vi "Old CAM Run Test.vi"() -> ()   [LabVIEW 2015]
uses:
  <vilib>/rvi/interface/nirviOpenFPGA/nirviOpenFPGA.xnode
  <vilib>/rvi/interface/nirviReadWriteControl/nirviReadWriteControl.xnode
  <vilib>/rvi/interface/Simulation/niFpgaSimulationCallBeginRW.vi
  <vilib>/rvi/errors/niLvFpgaAdjustHostInterfaceError.vi
  <vilib>/rvi/interface/nirviMethod/nirviMethod.xnode
  <vilib>/rvi/interface/nirviCloseFPGA/nirviCloseFPGA.xnode
  NiFpgaLv.dll
  <vilib>/Utility/error.llb/Error Cluster From Error Code.vi
  Compile Tests/old APU + 4 CAMs.vi
  <vilib>/rvi/interface/RandomDataEmulation/nirviRandomDataOpen.vi
  <vilib>/rvi/interface/common/niFpgaCacheSessionInfoDynamic.vi
  <vilib>/FPGAPlugInAG/Dynamic/niLvFpga_Run_Dynamic.vi
  <vilib>/FPGAPlugInAG/Dynamic/niLvFpga_Close_Dynamic.vi
  Data File Loader/AngleReference.ctl
panel:
  in  "Tooth Angles":cluster{"Falling Edge":dbl, "Rising Edge":dbl}[](array[cluster])=[{"Falling Edge"=0.0, "Rising Edge"=360.0}]
  out "Load done":bool
  out "Load time (s)":dbl=1.2129865353927016e-05
  in  "RPM":dbl=500.0 format="%#_15g"
  in  "stop":bool
  in  "acceleration (RPM/sec)":dbl=inf
  in  "CycleAngle?":T1=TRUE
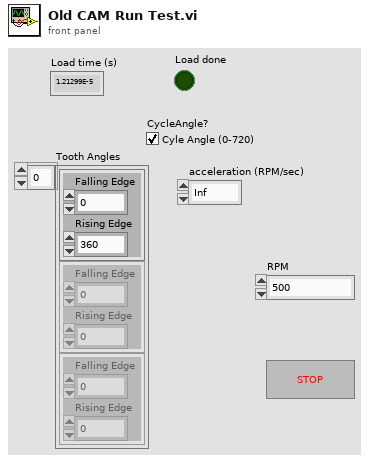
[diagram p1: front panel]
types:
  T1 = typedef "AngleReference.ctl" = bool
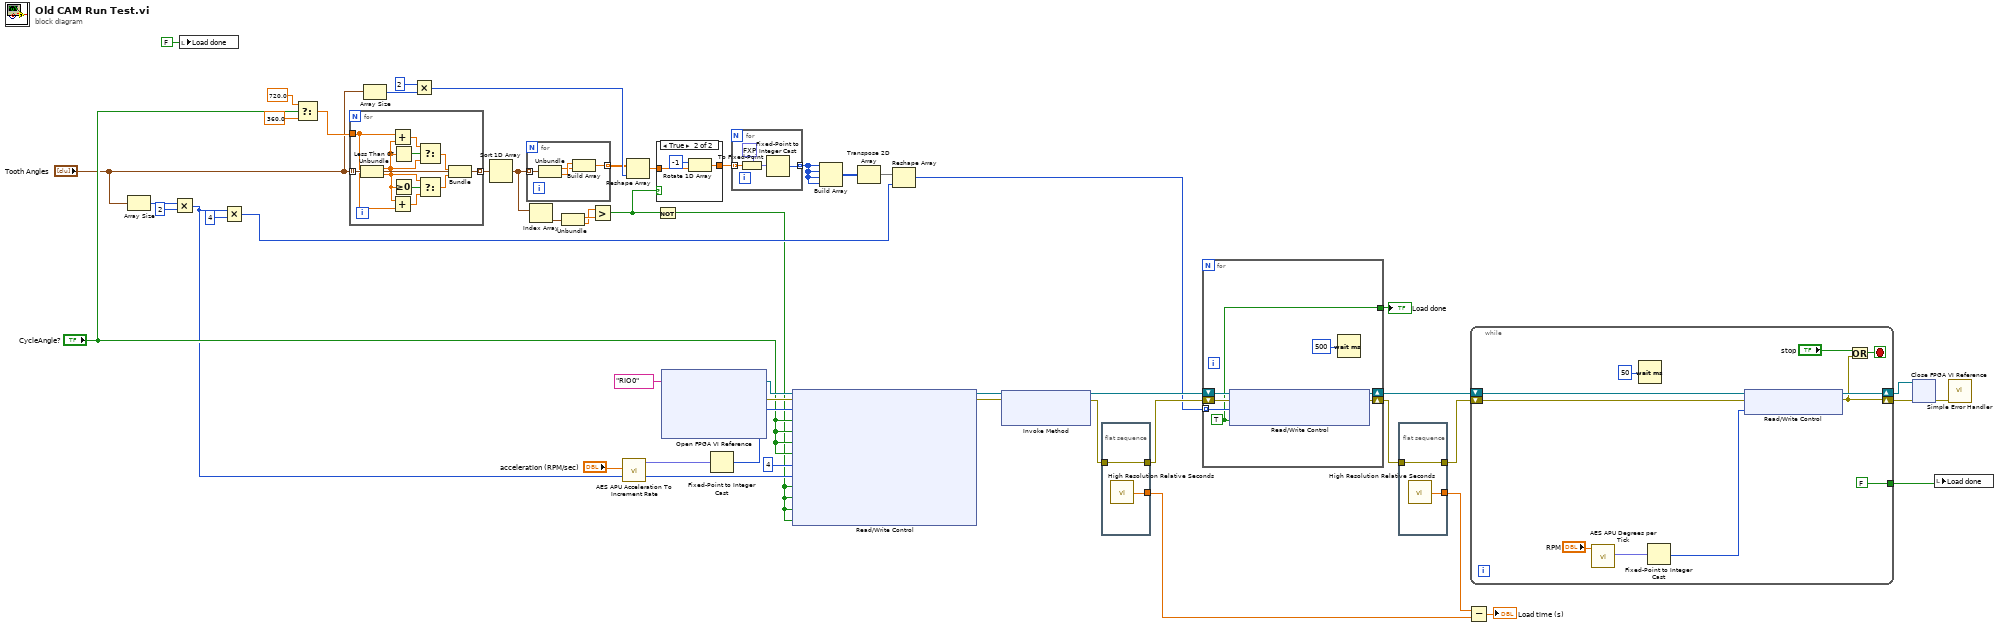
[diagram p0: block diagram]
diagram:
  n1 = Array Size(array="Tooth Angles") -> (size(s)=w11:i32)
  n2 = Multiply(x=w11, y=2) -> (x*y=w6:i32)
  n3 = local write "Load done"(FALSE ("Load done")) -> ()
  n4 = Multiply(x=w6, y=4) -> (x*y=w4:i32)
  n5 = Select(t=720.0 ("y"), s="CycleAngle?", f=360.0) -> (s? t:f=w16:dbl)
  n6 = for {
    tunnel: "Tooth Angles" -> [w56] mode=indexing
    tunnel: [w53] -> w19 mode=indexing
    tunnel: w16 -> [w52]
    n7 = Unbundle(w56) -> ("Falling Edge"=w59:dbl, "Rising Edge"=w57:dbl)
    n8 = Add(x=w52, y=w59) -> (x+y=w60:dbl)
    n9 = Add(x=w57, y=w52) -> (x+y=w58:dbl)
    n10 = Less Than 0?(x=w59) -> (x < 0?=w62:bool)
    n11 = Greater Or Equal To 0?(x=w57) -> (x >= 0?=w61:bool)
    n12 = Select(t=w60, s=w62, f=w59) -> (s? t:f=w55:dbl)
    n13 = Select(t=w57, s=w61, f=w58) -> (s? t:f=w54:dbl)
    n14 = Bundle(cluster=w56, "Falling Edge"=w55, "Rising Edge"=w54) -> (w53:cluster{"Falling Edge":dbl, "Rising Edge":dbl})
  }
  n15 = Array Size(array="Tooth Angles") -> (size(s)=w28:i32)
  n16 = Multiply(x=u16 2, y=w28) -> (x*y=w29:i32)
  n17 = Sort 1D Array(array=w19) -> (sorted array=w21:cluster{"Falling Edge":dbl, "Rising Edge":dbl}[])
  n18 = for {
    tunnel: w21 -> [w66] mode=indexing
    tunnel: [w63] -> w20 mode=indexing
    n19 = Unbundle(w66) -> ("Falling Edge"=w64:dbl, "Rising Edge"=w65:dbl)
    n20 = Build Array(w65, w64) -> (w63:dbl[])
  }
  n21 = Index Array(array=w21) -> (element=w22:cluster{"Falling Edge":dbl, "Rising Edge":dbl})  [unwired: 1 in]
  n22 = Unbundle(w22) -> ("Falling Edge"=w24:dbl, "Rising Edge"=w23:dbl)
  n23 = Greater?(x=w23, y=w24) -> (0:w26:bool)
  n24 = call <userlib>:"AES APU Acceleration To Increment Rate.vi"("acceleration (RPM/sec)"="acceleration (RPM/sec)") -> ("increment rate"=w31:fxp<+/-,47,-4>)  [unwired: 10 in]
  n25 = Reshape Array(w20, w29) -> (w25:dbl[])
  n26 = case shown="True" w26 {
    tunnel: w25 -> [w67 w70]
    tunnel: [w67 w68] -> w18
    frame False {
    }
    frame True {
      n27 = Rotate 1D Array(1:w70, 2:-1 ("n")) -> (0:w68:dbl[])
    }
  }
  n28 = Not(x=w26) -> (.not. x?=w3:bool)
  n29 = xnode "Open FPGA VI Reference"("resource name"=tag "RIO0") -> ("FPGA VI Reference Out"=w35:refnum<k20>, "error out"=w48:errorcluster)  [unwired: 1 in]
  n30 = Fixed-Point to Integer Cast(1:w31) -> (0:w30:i64)
  n31 = for {
    tunnel: w18 -> [w74] mode=indexing
    tunnel: [w71] -> w8 mode=indexing
    n32 = To Fixed-Point(fixed-point type=fxp<+,61,10> 0.0 ("Element"), number=w74) -> (fixed-point=w72:fxp<+,61,10>)
    n33 = Fixed-Point to Integer Cast(1:w72) -> (0:w71:u64)
  }
  n34 = xnode "Read/Write Control"("FPGA VI Reference In"=w35, "error in"=w48, "APU.Increment Rate"=w30, "FullyCustomTeeth.Cams.Cam4.CycleAngle"="CycleAngle?", "FullyCustomTeeth.Cams.Cam3.CycleAngle"="CycleAngle?", "FullyCustomTeeth.Cams.Cam2.CycleAngle"="CycleAngle?", "FullyCustomTeeth.Cams.Cam1.CycleAngle"="CycleAngle?", "FullyCustomTeeth.Cams.Num Profiles"=u8 4, "FullyCustomTeeth.Cams.Num Angles"=w6, "FullyCustomTeeth.Cams.Cam1.First Rising?"=w3, "FullyCustomTeeth.Cams.Cam2.First Rising?"=w3, "FullyCustomTeeth.Cams.Cam3.First Rising?"=w3, "FullyCustomTeeth.Cams.Cam4.First Rising?"=w3) -> ("FPGA VI Reference Out"=w43:refnum<k20>, "error out"=w34:errorcluster)
  n35 = Build Array(w8, w8, w8, w8) -> (w7:u64[][])
  n36 = Transpose 2D Array(2D array=w7) -> (transposed array=w9:u64[][])
  n37 = Reshape Array(w9, w4) -> (w2:u64[])
  n38 = xnode "Invoke Method"("FPGA VI Reference In"=w43, "error in"=w34) -> ("FPGA VI Reference Out"=w42:refnum<k20>, "error out"=w40:errorcluster)  [unwired: 1 in]
  n39 = flat-sequence {
    tunnel: [w76] -> w41
    tunnel: w40 -> [w76]
    tunnel: [w75] -> w38
    frame #0 {
      n40 = call <vilib>:"High Resolution Relative Seconds.vi"() -> ("relative seconds"=w75:dbl)
    }
  }
  n41 = for {
    shift-right: [w81] -> w33
    shift-left: w41 -> [w83]
    shift-right: [w80] -> w36
    shift-left: w42 -> [w82]
    tunnel: w2 -> [w79] mode=indexing
    tunnel: [w78] -> w1
    w78 = TRUE ("Done")
    n42 = xnode "Read/Write Control"("FPGA VI Reference In"=w82, "error in"=w83, "FullyCustomTeeth.Cams.Data"=w79, "FullyCustomTeeth.Cams.Toggle"=w78) -> ("FPGA VI Reference Out"=w80:refnum<k20>, "error out"=w81:errorcluster)
    n43 = Wait (ms)(milliseconds to wait=u32 500) -> ()  [unwired: 1 out]
  }
  "Load done" <- w1
  n44 = flat-sequence {
    tunnel: [w85] -> w32
    tunnel: w33 -> [w85]
    tunnel: [w84] -> w39
    frame #0 {
      n45 = call <vilib>:"High Resolution Relative Seconds.vi"() -> ("relative seconds"=w84:dbl)
    }
  }
  n46 = Subtract(x=w39, y=w38) -> (x-y=→"Load time (s)":dbl)
  n47 = while {
    shift-right: [w90] -> w51
    shift-left: w32 -> [w96]
    shift-right: [w94] -> w50
    shift-left: w36 -> [w95]
    tunnel: [FALSE ("Load")] -> w45
    stop <- w91 stop-if-true
    n48 = call <userlib>:"AES APU Degrees per Tick.vi"("RPM"="RPM") -> ("degrees per tick"=w87:fxp<+/-,47,-4>)  [unwired: 9 in, 1 out]
    n49 = Wait (ms)(milliseconds to wait=u32 50) -> ()  [unwired: 1 out]
    n50 = Fixed-Point to Integer Cast(1:w87) -> (0:w86:i64)
    n51 = xnode "Read/Write Control"("FPGA VI Reference In"=w95, "error in"=w96, "APU.Degrees per Tick"=w86) -> ("FPGA VI Reference Out"=w94:refnum<k20>, "error out"=w90:errorcluster)
    n52 = Or(x="stop", y=w90) -> (x .or. y?=w91:bool)
  }
  n53 = xnode "Close FPGA VI Reference"("FPGA VI Reference In"=w50, "error in"=w51) -> ("error out"=w49:errorcluster)
  n54 = local write "Load done"(w45) -> ()
  n55 = call <vilib>:"Simple Error Handler.vi"("error in (no error)"=w49) -> ()  [unwired: 4 in, 5 out]
